vi "Create Buffers.vi"(7 "framework configuration":T1, 8 "error in (no error)":errorcluster, 11 "Framework in":refnum<class "Framework.lvclass">) -> (0 "error out":errorcluster, 3 "Framework out":refnum<class "Framework.lvclass">)   [LabVIEW 2017, in "DSF Core.lvlib" / "Framework.lvclass"]
uses:
  Framework.lvclass
  Typedefs/DSF Engine Framework Configuration.ctl
  Typedefs/DSF Engine Plugin Configuration.ctl
  Typedefs/DSF Timing Info.ctl
  Typedefs/DSF Engine Plugin Thread Configuration.ctl
  Typedefs/DSF Settings Info.ctl
  Typedefs/DSF Engine Transfer Group Configuration.ctl
  Typedefs/DSF Direction.ctl
  Typedefs/DSF Engine Transfer Configuration.ctl
  Typedefs/DSF Byte Order.ctl
  Typedefs/DSF Engine Channel Configuration.ctl
  Typedefs/DSF Data Type.ctl
  Typedefs/DSF Timeout Behavior.ctl
  Buffer/Buffer.lvclass
  C:/Program Files (x86)/National Instruments/LabVIEW 2017/vi.lib/NI/Memory Manager/Classes/Pointer/Pointer.lvclass
  Framework.lvclass/Framework.ctl
  <vilib>/NI/Memory Manager/Classes/Pointer/Pointer.lvclass/Pointer.ctl
  <vilib>/NI/Memory Manager/Classes/Pointer/Set Size.vi
  <vilib>/NI/Memory Manager/Classes/Pointer/Set Address.vi
  <vilib>/NI/Memory Manager/Classes/Pointer/Check Null Pointer.vi
  <vilib>/NI/Memory Manager/Classes/Pointer/Set Internal.vi
  <vilib>/NI/Memory Manager/Classes/Pointer/Clear (No Check).vi
  <vilib>/NI/Memory Manager/Classes/Pointer/Check Length.vi
  <vilib>/NI/Memory Manager/Classes/Pointer/Errors.vi
  <vilib>/NI/Memory Manager/Classes/Pointer/Null Pointer.vi
  <vilib>/NI/Memory Manager/Classes/Pointer/Is Null.vi
  <vilib>/NI/Memory Manager/Classes/Pointer/Get Address.vi
  <vilib>/NI/Memory Manager/Classes/Pointer/Get Size.vi
  <vilib>/NI/Memory Manager/Classes/Pointer/Check Bounds (Pointer).vi
  <vilib>/NI/Memory Manager/Classes/Pointer/Create Error.vi
  <vilib>/NI/Memory Manager/Classes/Pointer/Out of Bounds.vi
  <vilib>/NI/Memory Manager/Constants/Constants.vi
  <vilib>/NI/Memory Manager/Constants/Library Name.vi
  <vilib>/NI/Memory Manager/Classes/Pointer/Pointer Error Info.vi
  <vilib>/NI/Memory Manager/Constants/Pointer Class Name.vi
  <vilib>/NI/Memory Manager/Classes/Pointer/Write Pointer Size to Error.vi
  Configuration/Required Buffer Size (Framework).vi
  <vilib>/NI/Memory Manager/VIs/New Error Cluster.vi
  <vilib>/NI/Memory Manager/VIs/New Error Cluster (512B).vi
  <vilib>/NI/Memory Manager/VIs/Set Error Status.vi
  <vilib>/NI/Memory Manager/VIs/Set Error Code.vi
  <vilib>/NI/Memory Manager/VIs/Set Error Source.vi
  <vilib>/NI/Memory Manager/VIs/Write String to Source.vi
  <vilib>/NI/Memory Manager/VIs/Write Numeric to Source.vi
  <vilib>/NI/Memory Manager/VIs/Write Numeric Scalar to Source (Base10 U64).vi
  Buffers/Buffers.lvclass
  Configuration/Configuration Session.lvclass
  <vilib>/NI/Memory Manager/Classes/Pointer/Pointer.lvclass
  DSF Core.lvlib
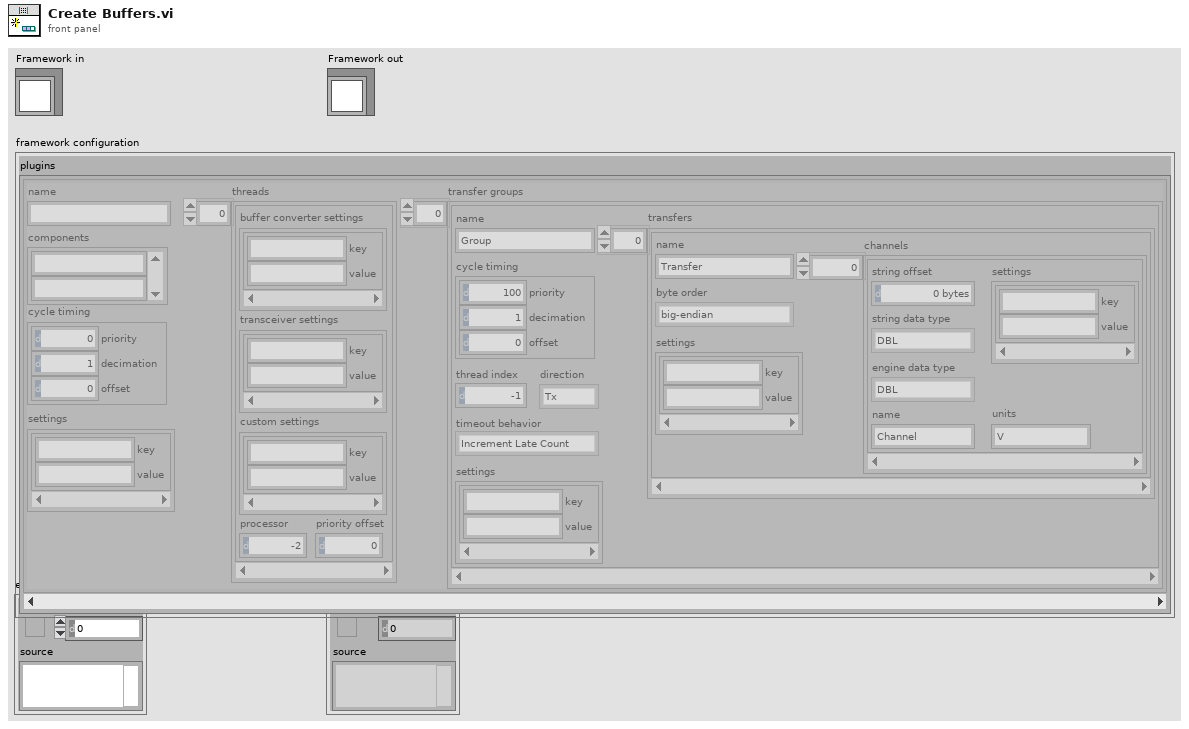
[diagram p1: front panel]
types:
  T1 = typedef "DSF Core.lvlib/DSF Engine Framework Configuration.ctl" = cluster{"plugins":T2[]}
  T2 = typedef "DSF Core.lvlib/DSF Engine Plugin Configuration.ctl" = cluster{"name":string, "components":string[], "cycle timing":T3, "threads":T4[], "transfer groups":T6[], "settings":T5}
  T3 = typedef "DSF Core.lvlib/DSF Timing Info.ctl" = cluster{"priority":u64, "decimation":u64, "offset":u64}
  T4 = typedef "DSF Core.lvlib/DSF Engine Plugin Thread Configuration.ctl" = cluster{"buffer converter settings":T5, "transceiver settings":T5, "custom settings":T5, "processor":i32, "priority offset":i16}
  T5 = typedef "DSF Core.lvlib/DSF Settings Info.ctl" = cluster{"key":string, "value":string}[]
  T6 = typedef "DSF Core.lvlib/DSF Engine Transfer Group Configuration.ctl" = cluster{"name":string, "direction":T7, "cycle timing":T3, "thread index":i32, "settings":T5, "transfers":T8[], "timeout behavior":T12}
  T7 = typedef "DSF Core.lvlib/DSF Direction.ctl" = enum8{"Tx", "Rx"}
  T8 = typedef "DSF Core.lvlib/DSF Engine Transfer Configuration.ctl" = cluster{"name":string, "byte order":T9, "settings":T5, "channels":T10[]}
  T9 = typedef "DSF Core.lvlib/DSF Byte Order.ctl" = enum8{"big-endian", "little-endian"}
  T10 = typedef "DSF Core.lvlib/DSF Engine Channel Configuration.ctl" = cluster{"string offset":u64, "string data type":T11, "engine data type":T11, "name":string, "settings":T5, "units":string}
  T11 = typedef "DSF Core.lvlib/DSF Data Type.ctl" = enum8{"Bool", "SGL", "DBL", "I8", "I16", "I32", "I64", "U8", "U16", "U32", "U64"}
  T12 = typedef "DSF Core.lvlib/DSF Timeout Behavior.ctl" = enum8{"Increment Late Count", "Throw Error"}
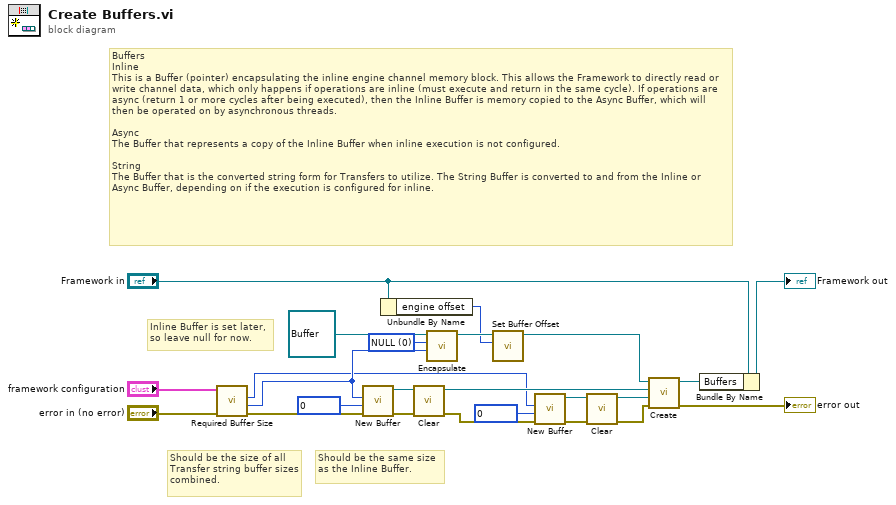
[diagram p0: block diagram]
diagram:
  w11 = u64 0 items=["NULL"] ("Null")
  # "Should be the size of all Transfer string buffer sizes combined."
  # "Should be the same size as the Inline Buffer."
  # "Buffers\nInline\nThis is a Buffer (pointer) encapsulating the inline engine channel memory block. This allows the Framework to directly read or write channel data, which only happens if operations are inline (must execute and return in the same cycle). If operations are async (return 1 or more cycles after being executed), then the Inline Buffer is memory copied to the Async Buffer, which will then be operated on by asynchronous threads.\n\nAsync\nThe Buffer that represents a copy of the Inline Buffer when inline execution is not configured.\n\nString\nThe Buffer that is the converted string form for Transfers to utilize. The String Buffer is converted to and from the Inline or Async Buffer, depending on if the execution is configured for inline."
  # "Inline Buffer is set later, so leave null for now."
  n1 = call-poly "Required Buffer Size.vi"("error in (no error)"="error in (no error)", "Framework Configuration in"="framework configuration") -> ("error out"=w21:errorcluster, "total engine buffer size"=w13:u64, "total string buffer size"=w2:u64)  [unwired: 6 in, 1 out]
  n2 = call "New Buffer.vi"("error in (no error)"=w21, "buffer offset (0)"=u64 0 ("buffer offset"), "buffer size"=w13) -> ("error out"=w8:errorcluster, "Buffer out"=w9:refnum<class "Buffer.lvclass">)  [unwired: 7 in]
  n3 = Unbundle By Name("Framework in") -> ("engine offset"=w12:u64)
  n4 = call <vilib>:"Clear.vi"("error in (no error)"=w8, "Pointer in"=w9) -> ("error out"=w7:errorcluster, "Pointer out"=w6:refnum<class "Buffer.lvclass">)  [unwired: 8 in]
  n5 = call <vilib>:"Encapsulate.vi"("size"=w13, "address"=w11, "Pointer type"=refnum<class "Buffer.lvclass"> refnum ("Inline Buffer (null)")) -> ("Pointer"=w14:refnum<class "Buffer.lvclass">)  [unwired: 7 in, 1 out]
  n6 = call "Set Buffer Offset.vi"("buffer offset"=w12, "Buffer in"=w14) -> ("Buffer out"=w10:refnum<class "Buffer.lvclass">)  [unwired: 9 in]
  n7 = call "New Buffer.vi"("error in (no error)"=w7, "buffer offset (0)"=u64 0 ("buffer offset"), "buffer size"=w2) -> ("error out"=w4:errorcluster, "Buffer out"=w5:refnum<class "Buffer.lvclass">)  [unwired: 7 in]
  n8 = call <vilib>:"Clear.vi"("error in (no error)"=w4, "Pointer in"=w5) -> ("error out"=w3:errorcluster, "Pointer out"=w1:refnum<class "Buffer.lvclass">)  [unwired: 8 in]
  n9 = call "Create.vi"("error in (no error)"=w3, "String Buffer (null)"=w1, "Async Buffer (null)"=w6, "Inline Buffer (null)"=w10) -> ("error out"=→"error out":errorcluster, "Buffers out"=w24:refnum<class "Buffers.lvclass">)  [unwired: 6 in]
  n10 = Bundle By Name(cluster="Framework in", "Buffers"=w24) -> (→"Framework out":refnum<class "Framework.lvclass">)
